vi "AUTO_HOME.vi"(8 "error in (no error)":errorcluster) -> (0 "error out":errorcluster)   [LabVIEW 2017]
doc: "This vi is for manually turn ON and OFF also monitor Output of PLCS. So this is manual screen."
uses:
  <vilib>/Utility/miscctls.llb/LVRowAndColumnUnsignedTypeDef.ctl
  8ff177a1-7a64-42a7-ac4f-5dbd57cfe52d.vi
  b56ad881-f772-481a-9ad8-33fdffb2c092.vi
  Global/PLC_to_Auto.vi
  <vilib>/Utility/file.llb/Read Delimited Spreadsheet (string).vi
  <vilib>/Utility/file.llb/Write Delimited Spreadsheet (string).vi
panel:
  out "Table":string[][](table)
  out "CYCLE STATUS 9":bool
  out "AUTO\nHOME STOP":bool
  in  "SPRING ABORT":bool
  in  "SPRING ACK":bool
  out "PART OK":bool
  out "SYSTEM READY":bool
  out "HAUSING STATUS":bool
  out "MAGNETIC STATUS":bool
  out "CBCT STATUS":bool
  out "PMR STATUS":bool
  out "KINEMATIC STATUS":bool
  out "KITTING ST NG COUNTER":u16 format="NG COUNTER: %.0f"
  out "KITTING ST OK COUNTER":u16 format="OK COUNTER: %.0f"
  out "KITTING ST CYCLE TIME":dbl format="CYCLE TIME : %.1f SEC"
  out "CYCLE STATUS 10":bool
  out "CYCLE STATUS 8":bool
  out "CYCLE STATUS 4":bool
  out "CYCLE STATUS 7":bool
  out "CYCLE STATUS 3":bool
  out "CYCLE STATUS 6":bool
  out "CYCLE STATUS 2":bool
  out "CYCLE STATUS 5":bool
  out "CYCLE STATUS 1":bool
  out "CYCLE TIME IN SEC":T1 {"CYCLE TIME 28" format="%.2f"; "CYCLE TIME 10" format="%.2f"; "CYCLE TIME 8" format="%.2f"; "CYCLE TIME 4" format="%.2f"; "CYCLE TIME 7" format="%.2f"; "CYCLE TIME 3" format="%.2f"; "CYCLE TIME 6" format="%.2f"; "CYCLE TIME 2" format="%.2f"; "CYCLE TIME 5" format="%.2f"; "CYCLE TIME 1" format="%.2f"}
  out "Plan Selected:":string
  out "USER:-":string
  out "ALARM Indicator":string
  out "DATE/TIME":string
  in  "Back":bool
  # "KITTING STATION - RCBO 2P2M"
  # "4.NEUTRAL\nIA ASSEMBLY"
  # "9.RIVITING\nSTATION"
  # "8.NEUTRAL\n2C ASSEMBLY"
  # "7.NEUTRAL\n2B ASSEMBLY"
  # "6.NEUTRAL\n2A ASSEMBLY"
  # "5.NEUTRAL\nIB ASSEMBLY"
  # "3.PHASE SIDE\nII ASSEMBLY"
  # "10.FINAL\nVISION SYSTEM"
  # "2.PHASE SIDE\nI ASSEMBLY"
  # "1.KITTING \nSTATION"
  # "CYCLE TIME IN SEC"
  # "OK COUNTER"
  # "NG COUNTER"
  # "CYCLE STATUS"
  # "ALARM:-"
  # "STATUS OF\n KITTING STATION"
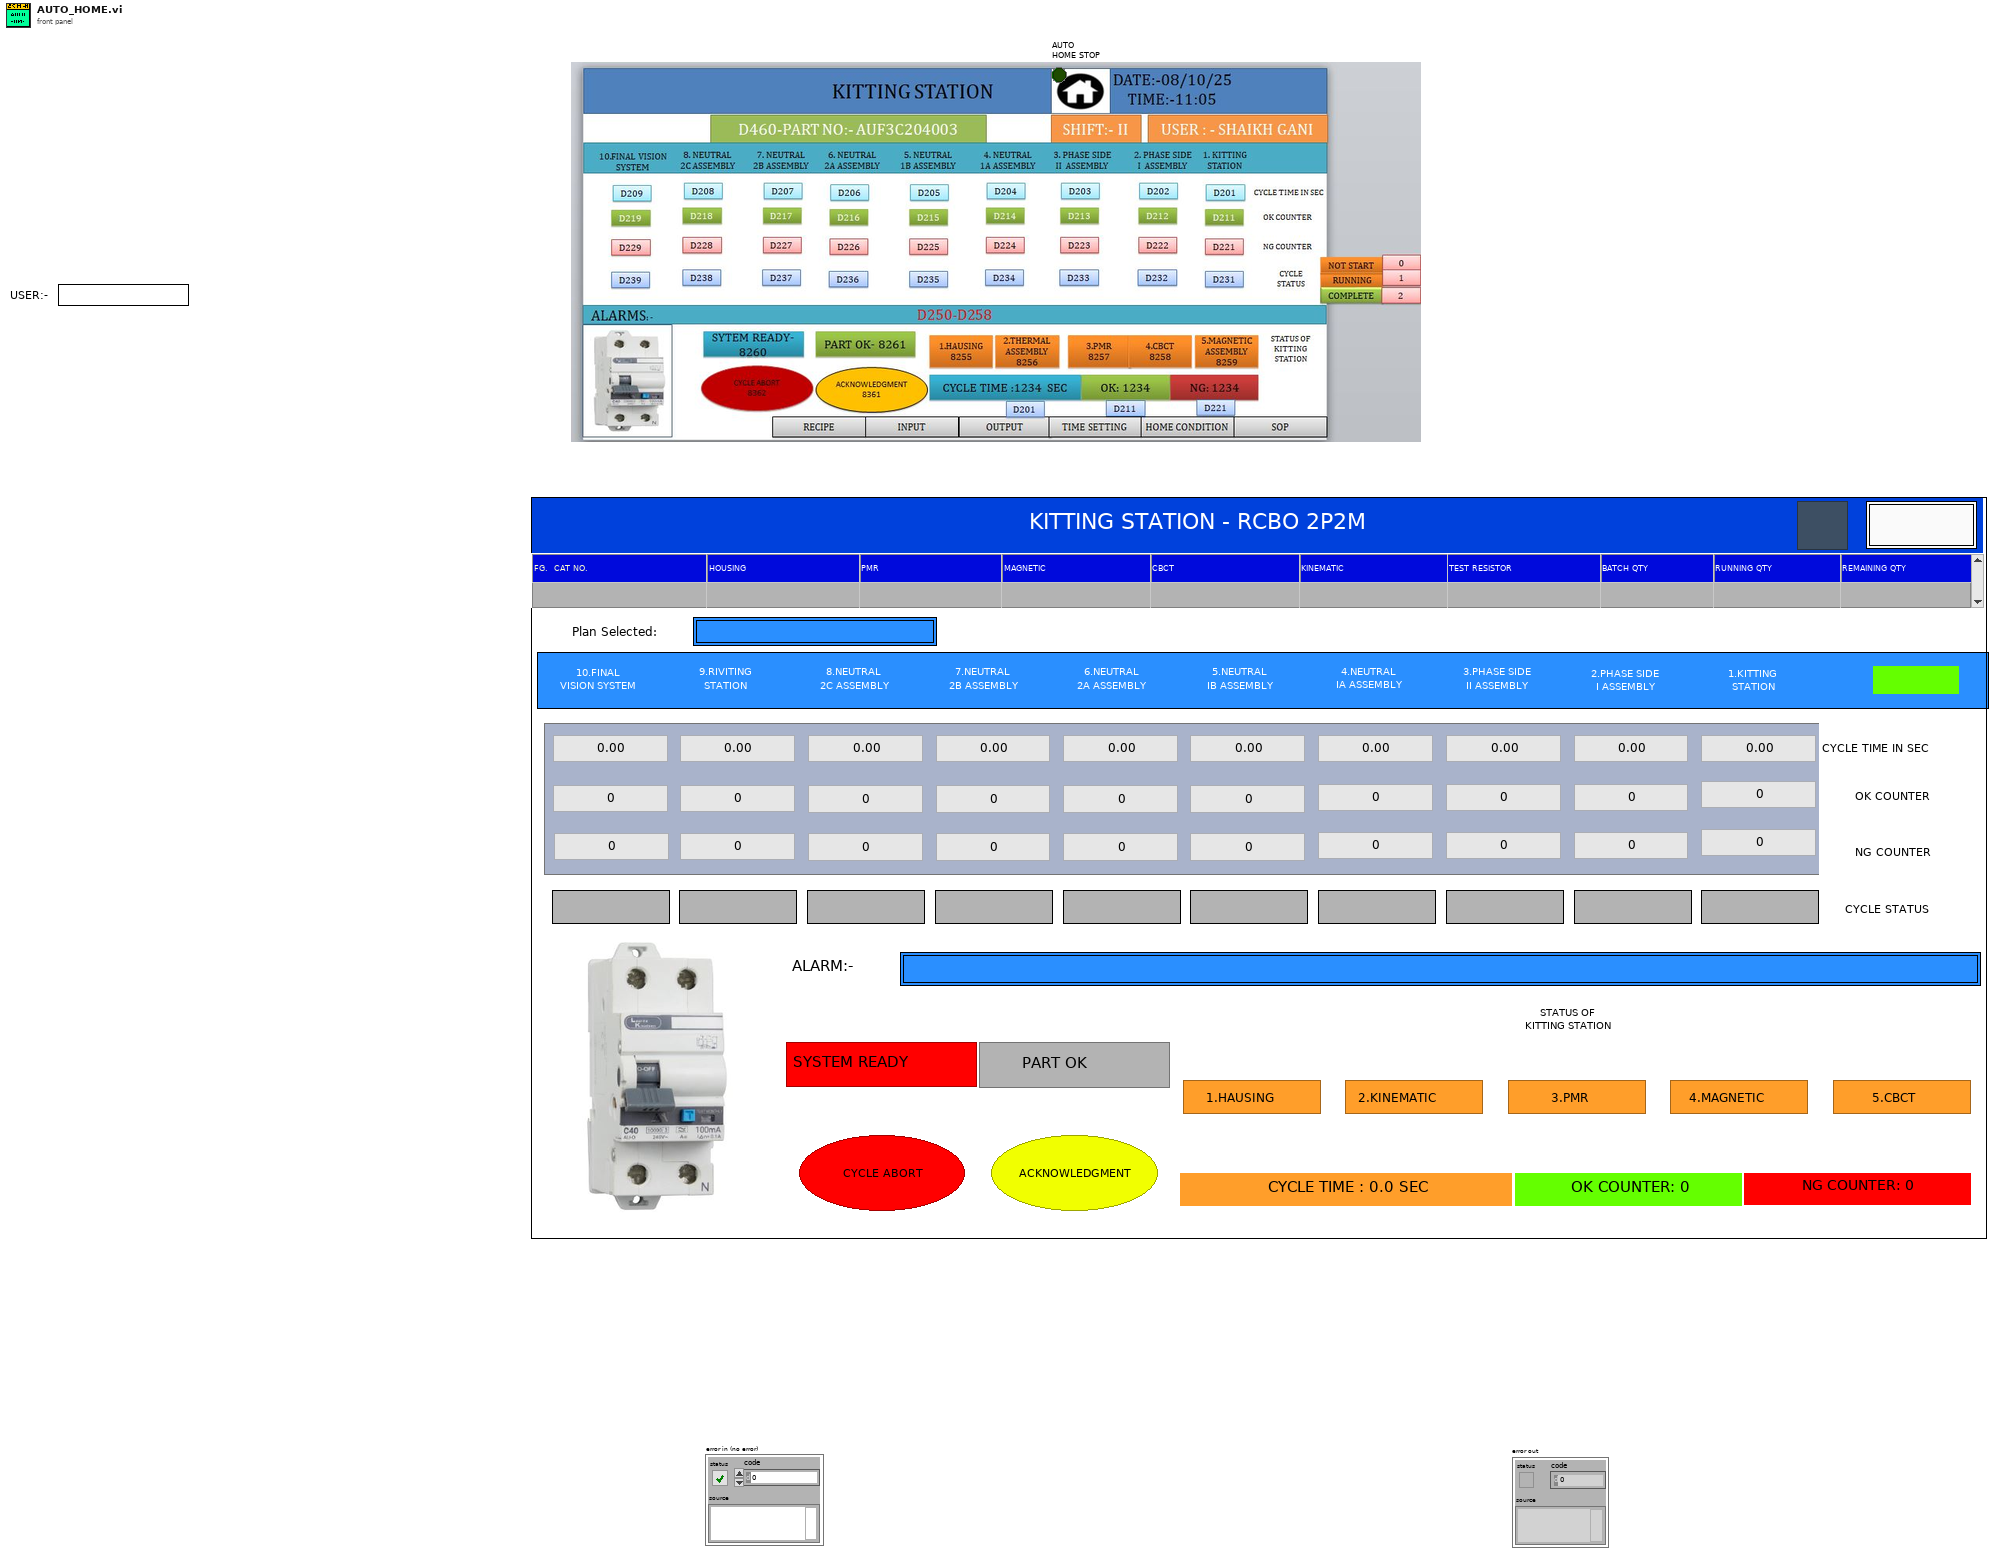
[diagram p1: front panel]
types:
  T1 = cluster{"[0]":dbl, "[1]":dbl, "[2]":dbl, "[3]":dbl, "[4]":dbl, "[5]":dbl, "[6]":dbl, "[7]":dbl, "[8]":dbl, "[9]":dbl, "CYCLE TIME 9":u16, "CYCLE TIME 12":u16, "CYCLE TIME 14":u16, "CYCLE TIME 16":u16, "CYCLE TIME 11":u16, "CYCLE TIME 13":u16, "CYCLE TIME 15":u16, "CYCLE TIME 17":u16, "CYCLE TIME 29":u16, "CYCLE TIME 18":u16, "CYCLE TIME 19":u16, "CYCLE TIME 21":u16, "CYCLE TIME 23":u16, "CYCLE TIME 25":u16, "CYCLE TIME 20":u16, "CYCLE TIME 22":u16, "CYCLE TIME 24":u16, "CYCLE TIME 26":u16, "CYCLE TIME 30":u16, "CYCLE TIME 27":u16}
  T2 = cluster{"SELECTED RECIPE":cluster{"TABLE":string[]}}
  T3 = typedef "LVRowAndColumnUnsignedTypeDef.ctl" = cluster{"Row":u32, "Column":u32}
  T4 = enum32{"invalid app kind", "Development System", "Run Time System", "Student Edition", "Embedded LabVIEW", "Evaluation", "Custom"}
  T5 = cluster{"[0]":dbl, "[1]":dbl, "[2]":dbl, "[3]":dbl, "[4]":dbl, "[5]":dbl, "[6]":dbl, "[7]":dbl, "[8]":dbl, "[9]":dbl, "[10]":dbl, "[11]":dbl, "[12]":dbl, "[13]":dbl, "[14]":dbl, "[15]":dbl, "[16]":dbl, "[17]":dbl, "[18]":dbl, "[19]":dbl, "[20]":dbl, "[21]":dbl, "[22]":dbl, "[23]":dbl, "[24]":dbl, "[25]":dbl, "[26]":dbl, "[27]":dbl, "[28]":dbl, "[29]":dbl}
  T6 = enum32{"Invalid", "Standard", "Closed", "Hidden", "Minimized", "Maximized"}
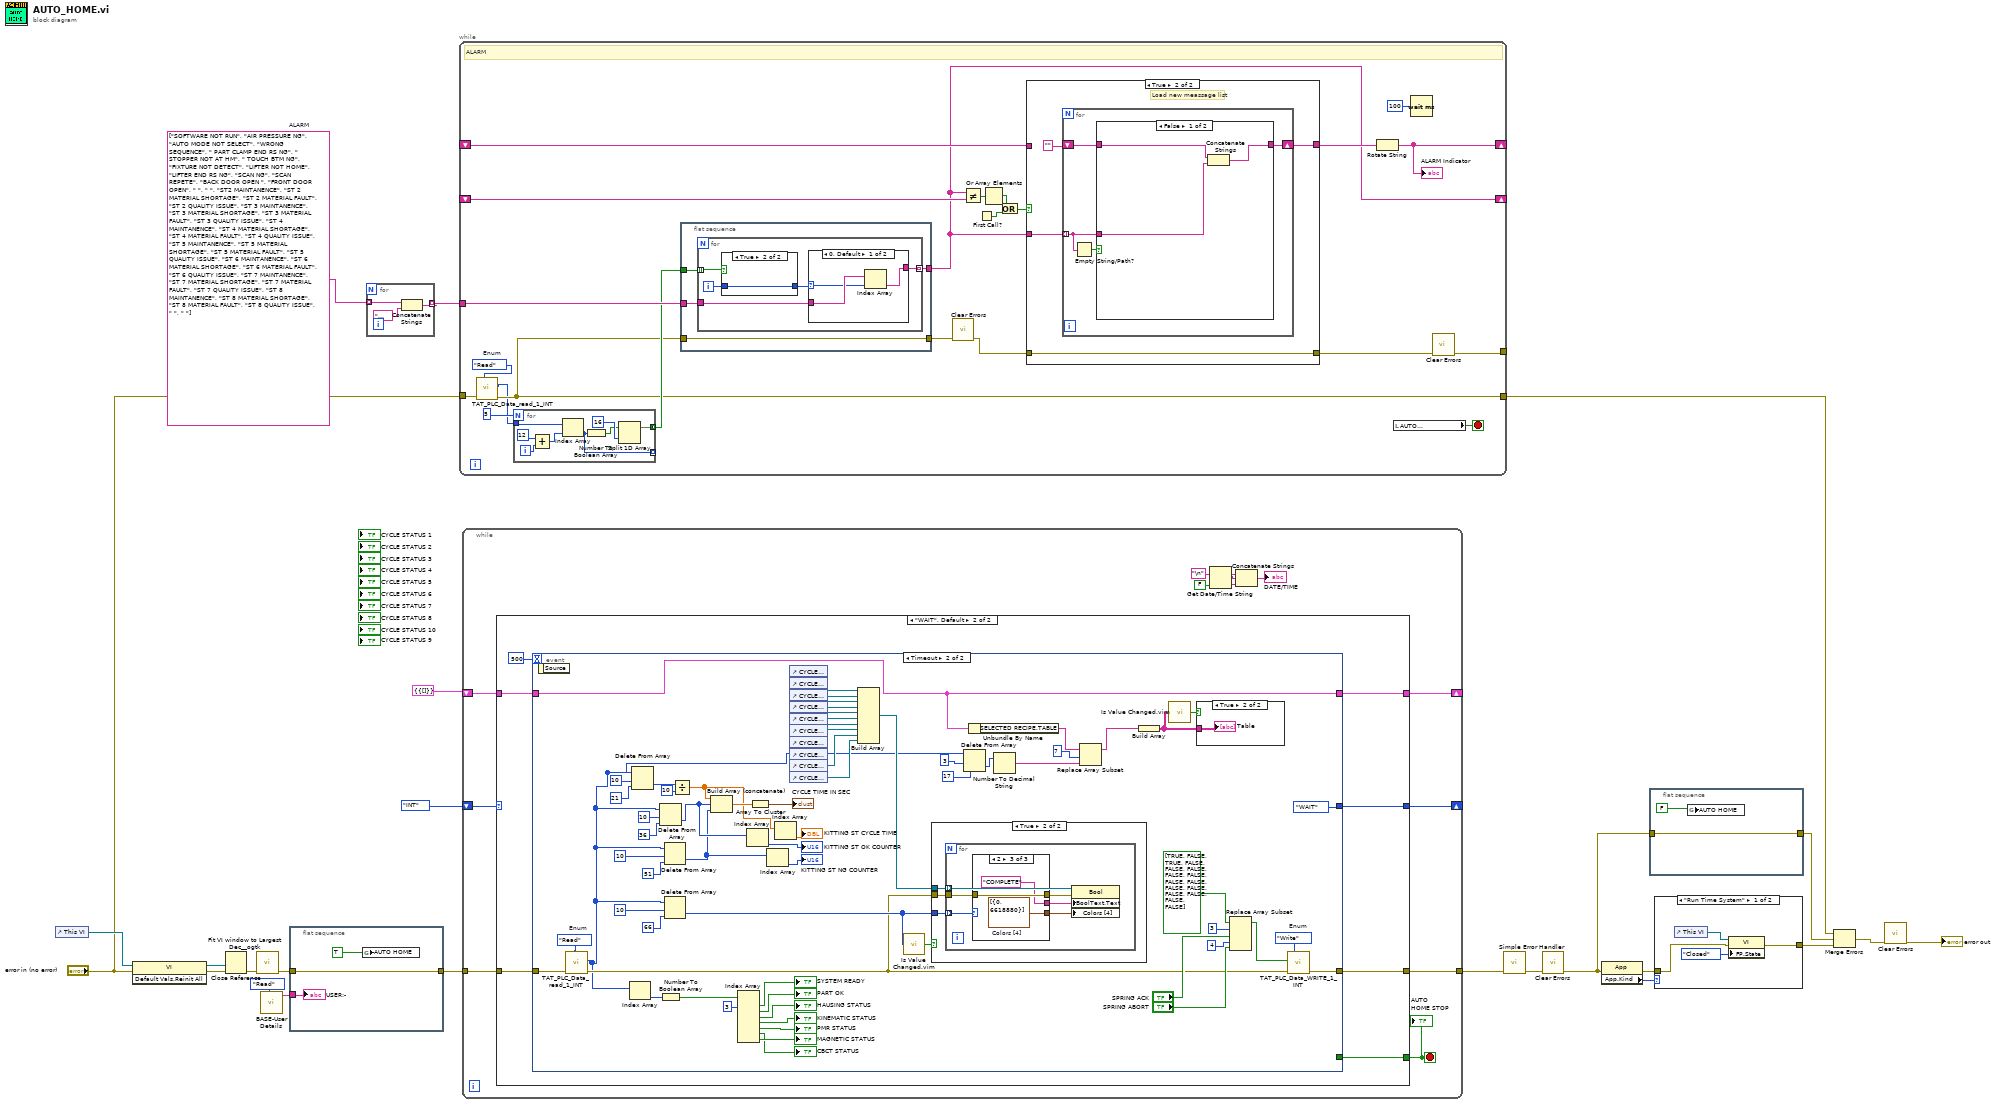
[diagram p0: block diagram]
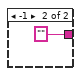
[diagram p2: hidden frame]
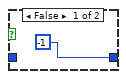
[diagram p3: hidden frame]
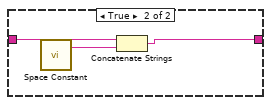
[diagram p5: hidden frame]
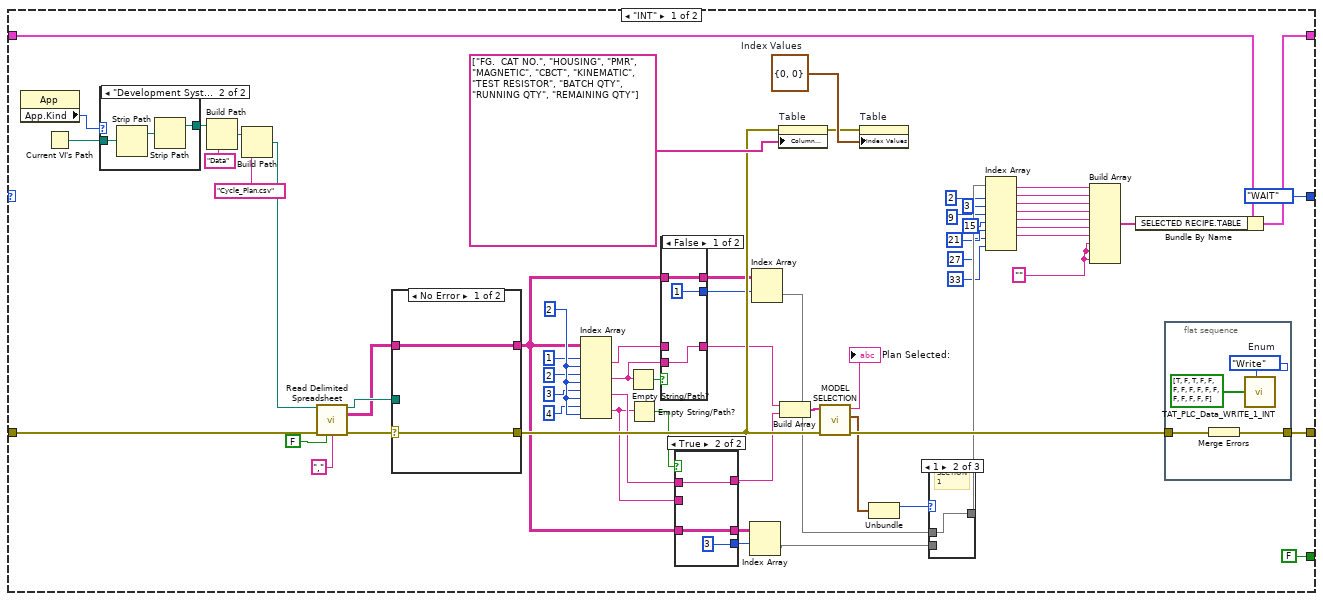
[diagram p7: hidden frame]
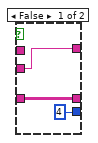
[diagram p10: hidden frame]
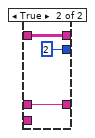
[diagram p11: hidden frame]
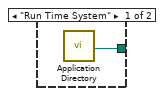
[diagram p12: hidden frame]
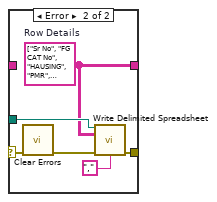
[diagram p13: hidden frame]
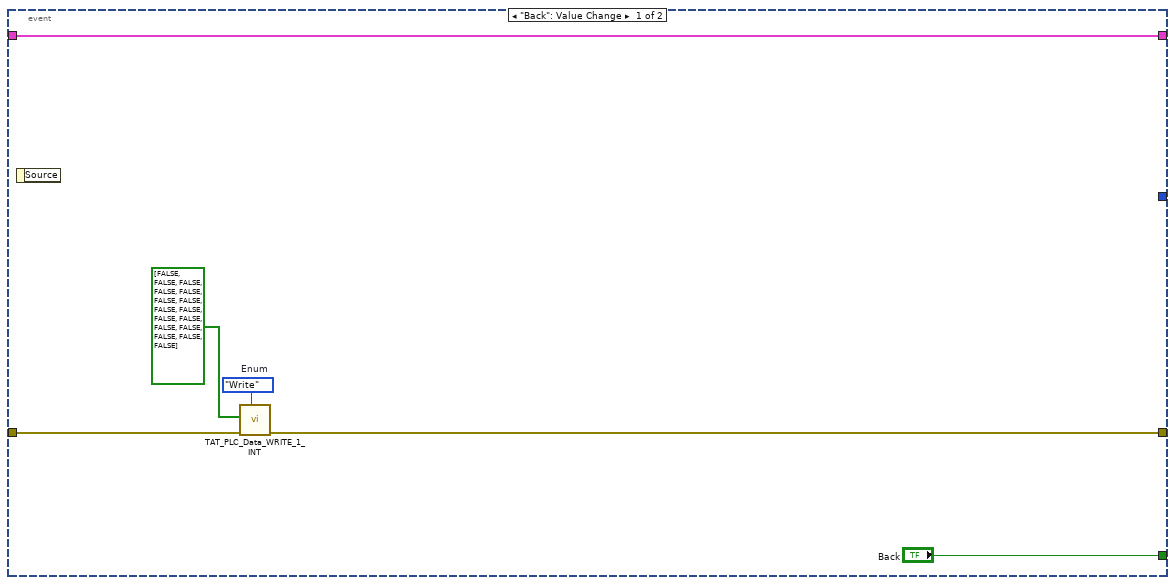
[diagram p14: hidden frame]
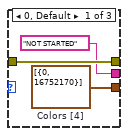
[diagram p17: hidden frame]
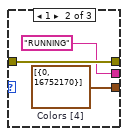
[diagram p18: hidden frame]
diagram:
  w2 = string[] ["SOFTWARE NOT RUN", "AIR PRESSURE NG", "AUTO MODE NOT SELECT", "WRONG SEQUENCE", " PART CLAMP END RS NG", " STOPPER NOT AT HM", " TOUCH BTM NG", "FIXTURE NOT DETECT", "LIFTER NOT HOME", "LIFTER END RS NG", "SCAN NG", "SCAN  REPETE", "BACK DOOR OPEN ", "FRONT DOOR OPEN", " ", " ", "ST2 MAINTANENCE", "ST 2 MATERIAL SHORTAGE", "ST 2 MATERIAL FAULT", "ST 2 QUALITY ISSUE", "ST 3 MAINTANENCE", "ST 3 MATERIAL SHORTAGE", "ST 3 MATERIAL FAULT", "ST 3 QUALITY ISSUE", "ST 4 MAINTANENCE", "ST 4 MATERIAL SHORTAGE", "ST 4 MATERIAL FAULT", "ST 4 QUALITY ISSUE", "ST 5 MAINTANENCE", "ST 5 MATERIAL SHORTAGE", "ST 5 MATERIAL FAULT", "ST 5 QUALITY ISSUE", "ST 6 MAINTANENCE", "ST 6 MATERIAL SHORTAGE", "ST 6 MATERIAL FAULT", "ST 6 QUALITY ISSUE", "ST 7 MAINTANENCE", "ST 7 MATERIAL SHORTAGE", "ST 7 MATERIAL FAULT", "ST 7 QUALITY ISSUE", "ST 8 MAINTANENCE", "ST 8 MATERIAL SHORTAGE", "ST 8 MATERIAL FAULT", "ST 8 QUALITY ISSUE", " ", " "]  # ALARM
  n1 = control-ref of="This VI"() -> (w19:refnum<vi>)
  n2 = invoke class="VI" method="Default Vals.Reinit All"(reference=w19, error in="error in (no error)") -> (reference out=w18:refnum<vi>, error out=w17:errorcluster)  [unwired: 1 in, 1 out]
  n3 = Close Reference(reference=w18, error in (no error)=w17) -> (error out=w16:errorcluster)
  n4 = call <userlib>:"Fit VI window to Largest Dec__ogtk.vi"("error in (no error)"=w16) -> ("error out"=w15:errorcluster)  [unwired: 5 in, 1 out]
  n5 = call "BASE-User Details.vi"("Enum"=enum16{"Read", "Write"}."Read") -> ("User Name Out"=w7:string)  [unwired: 9 in, 1 out]
  n6 = flat-sequence {
    tunnel: w15 -> [w26]
    tunnel: [w26] -> w11
    tunnel: w7 -> [w24]
    frame #0 {
      n7 = global write "PLC_to_Auto.vi" "AUTO HOME"(TRUE) -> ()
      "USER:-" <- w24
    }
  }
  n8 = for {
    tunnel: w2 -> [w29] mode=indexing
    tunnel: [w27] -> w5 mode=indexing
    n9 = Concatenate Strings(w29, "          ") -> (w27:string)
  }
  n10 = while {
    tunnel: "error in (no error)" -> [w33]
    tunnel: [w40] -> _
    tunnel: w5 -> [w38]
    shift-right: [w36] -> _
    shift-left: _ -> [w47]
    shift-right: [w46] -> _
    shift-left: _ -> [w48]
    tunnel: [w32] -> w3
    stop <- w37 stop-if-true
    w30 = enum16{"Read", "Write"}."Read"  # Enum
    # "ALARM"
    n11 = call "TAT_PLC_Data_read_1_INT.vi"("Enum"=w30, "error in (no error)"=w33) -> ("error out"=w32:errorcluster, "Array 2"=w31:u16[])  [unwired: 8 in]
    n12 = for {
      N: 5 -> [_]
      tunnel: w31 -> [w59]
      tunnel: [w53] -> w34 mode=concatenating
      tunnel: [w52] -> _ mode=indexing
      i -> [w57]
      n13 = Add(x=12, y=w57) -> (x+y=w56:i32)
      n14 = Index Array(array=w59, index=w56) -> (element=w52:u16)
      n15 = Number To Boolean Array(number=w52) -> (Boolean array=w54:bool[])
      n16 = Split 1D Array(array=w54, index=16) -> (first subarray=w53:bool[])  [unwired: 1 out]
    }
    n17 = flat-sequence {
      tunnel: [w61] -> w42
      tunnel: [w63] -> w46
      tunnel: w38 -> [w62]
      tunnel: w32 -> [w61]
      tunnel: w34 -> [w60]
      frame #0 {
        n18 = for {
          tunnel: w60 -> [w68] mode=indexing
          tunnel: [w64] -> w63 mode=indexing
          tunnel: w62 -> [w66]
          i -> [w67]
          n19 = case shown="True" w68 {
            tunnel: w67 -> [_ w74]
            tunnel: [-1 w74] -> w65
            frame False {
            }
            frame True {
            }
          }
          n20 = case shown="0, Default" w65 {
            selector: w65 -> [w70 _]
            tunnel: w66 -> [w71 _]
            tunnel: [w69 ""] -> w64
            frame 0, Default {
              n21 = Index Array(array=w71, index=w70) -> (element=w69:string)
            }
            frame -1 {
            }
          }
        }
      }
    }
    n22 = call <vilib>:"Clear Errors.vi"("error in (no error)"=w42) -> ("error out"=w41:errorcluster)  [unwired: 5 in, 1 out]
    n23 = Not Equal?(x=w46, y=w48) -> (x != y?=w50:bool[])
    n24 = First Call?() -> (First Call?: T/F=w45:bool)
    n25 = Or Array Elements(Boolean array=w50) -> (logical OR=w44:bool)
    n26 = Or(x=w44, y=w45) -> (x .or. y?=w43:bool)
    n27 = case shown="True" w43 {
      tunnel: [w76 w78] -> w49
      tunnel: w47 -> [w76 _]
      tunnel: w46 -> [_ w79]
      tunnel: w41 -> [w75 w77]
      tunnel: [w75 w77] -> w39
      frame False {
      }
      frame True {
        # "Load new meassage list"
        n28 = for {
          tunnel: w79 -> [w82] mode=indexing
          shift-right: [w84] -> w78
          shift-left: "" -> [w83]
          n29 = Empty String/Path?(string/path=w82) -> (empty?=w81:bool)
          n30 = case shown="False" w81 {
            tunnel: [w87 w90] -> w84
            tunnel: w83 -> [w86 w89]
            tunnel: w82 -> [w85 _]
            frame False {
              n31 = Concatenate Strings(w86, w85) -> (w87:string)
            }
            frame True {
              n32 = call <vilib>:"Space Constant.vi"() -> ("String"=w88:string)
              n33 = Concatenate Strings(w89, w88) -> (w90:string)
            }
          }
        }
      }
    }
    n34 = Rotate String(1:w49) -> (0:w36:string)
    "ALARM Indicator" <- w36
    n35 = local read "AUTO\nHOME STOP"() -> (w37:bool)
    n36 = Wait (ms)(milliseconds to wait=u32 100) -> ()  [unwired: 1 out]
    n37 = call <vilib>:"Clear Errors.vi"("error in (no error)"=w39) -> ("error out"=w40:errorcluster)  [unwired: 5 in, 1 out]
  }
  n38 = while {
    tunnel: w11 -> [w102]
    tunnel: [w101] -> w22
    shift-right: [w98] -> _
    shift-left: enum16{"INT", "WAIT"}."INT" -> [w99]
    shift-right: [w92] -> _
    shift-left: T2 {"SELECTED RECIPE"={"TABLE"=[]}} -> [w91]
    stop <- w100 stop-if-true
    n39 = case shown="\"WAIT\", Default" w99 {
      tunnel: w102 -> [w161 w203]
      tunnel: [w122 w202] -> w101
      tunnel: [FALSE w201] -> w100
      tunnel: [enum16{"INT", "WAIT"}."WAIT" w199] -> w98
      tunnel: [w104 w198] -> w92
      tunnel: w91 -> [w105 w197]
      frame "INT" {
        w113 = ""
        w146 = 2
        w148 = T3 {"Row"=0, "Column"=0}  # Index Values
        n40 = property class="App"() -> ("App.Kind"=w159:T4)  [unwired: 2 in, 2 out]
        n41 = Current VI's Path() -> (path=w160:path)
        n42 = case shown="\"Development System\", Default" w159 {
          tunnel: w160 -> [_ w187]
          tunnel: [w185 w186] -> w157
          frame "Run Time System" {
            n43 = call <vilib>:"Application Directory.vi"() -> ("Application Directory"=w185:path)
          }
          frame "Development System", Default {
            n44 = Strip Path(path=w187) -> (stripped path=w188:path)  [unwired: 1 out]
            n45 = Strip Path(path=w188) -> (stripped path=w186:path)  [unwired: 1 out]
          }
        }
        n46 = Build Path(base path=w157, name or relative path="Data") -> (appended path=w155:path)
        n47 = Build Path(base path=w155, name or relative path="Cycle_Plan.csv") -> (appended path=w154:path)
        n48 = call-poly <vilib>:"Read Delimited Spreadsheet.vi"("file path (dialog if empty)"=w154, "error in (no error)"=w161, "transpose? (F)"=FALSE, "delimiter (\\t)"=",") -> ("new file path (Not A Path if cancelled)"=w165:path, "all rows"=w164:string[][], "error out"=w166:errorcluster)  [unwired: 6 in, 3 out]
        n49 = case shown="No Error" w166 {
          selector: w166 -> [w190 w196]
          tunnel: [w190 w194] -> w149
          tunnel: w165 -> [_ w193]
          tunnel: [w189 w191] -> w126
          tunnel: w164 -> [w189 _]
          frame No Error {
          }
          frame Error {
            w191 = string[][] [["Sr No", "FG CAT No", "HAUSING", "PMR", "MAGNETIC ASLY", "CBCT GROUP", "KINEMATIC ASLY", "TEST RESISTOR"]]  # Row Details
            n50 = call <vilib>:"Clear Errors.vi"("error in (no error)"=w196) -> ("error out"=w195:errorcluster)  [unwired: 5 in, 1 out]
            n51 = call-poly <vilib>:"Write Delimited Spreadsheet.vi"("file path (dialog if empty)"=w193, "2D data"=w191, "error in (no error)"=w195, "delimiter (\\t)"=",") -> ("error out"=w194:errorcluster)  [unwired: 10 in, 1 out]
          }
        }
        n52 = Index Array(array=w126, index (row) #1=1, index (col) #1=w146, index (row) #2=2, index (col) #2=w146, index (row) #3=3, index (col) #3=w146, index (row) #4=4, index (col) #4=w146) -> (element #1=w140:string, element #2=w139:string, element #3=w137:string, element #4=w136:string)
        n53 = Empty String/Path?(string/path=w139) -> (empty?=w141:bool)
        n54 = Empty String/Path?(string/path=w136) -> (empty?=w138:bool)
        n55 = case shown="False" w141 {
          tunnel: w140 -> [_ w184]
          tunnel: w139 -> [w181 _]
          tunnel: [w181 w184] -> w135
          tunnel: w126 -> [w179 w183]
          tunnel: [1 2] -> w129
          tunnel: [w179 w183] -> w128
          frame False {
          }
          frame True {
          }
        }
        n56 = case shown="True" w138 {
          tunnel: w137 -> [_ w178]
          tunnel: w136 -> [w175 _]
          tunnel: [w175 w178] -> w130
          tunnel: w126 -> [w174 w176]
          tunnel: [w174 w176] -> w125
          tunnel: [4 3] -> w124
          frame False {
          }
          frame True {
          }
        }
        n57 = Index Array(array=w125, index (row)=w124) -> (element=w123:string[])  [unwired: 1 in]
        n58 = Index Array(array=w128, index (row)=w129) -> (element=w127:string[])  [unwired: 1 in]
        n59 = property on="Table" class="Tbl (strict)"(error in=w149, "Column Headers[]"=string[] ["FG.  CAT NO.", "HOUSING", "PMR", "MAGNETIC", "CBCT", "KINEMATIC", "TEST RESISTOR", "BATCH QTY", "RUNNING QTY", "REMAINING QTY"]) -> (error out=w147:errorcluster)  [unwired: 1 in, 1 out]
        n60 = Build Array(w135, w130) -> (w134:string[])
        n61 = call "MODEL SELECTION.vi"("error in (no error)"=w149, "Plan List"=w134) -> ("error out 2"=w152:errorcluster, "SELECTED RECIPE\nand COMBI OF BIN- INDEX"=w132:cluster{"RECIPE INDEX":i32, "COMBI BIN":i32}, "Plan Selected"=→"Plan Selected:":string)  [unwired: 7 in]
        n62 = property on="Table" class="Tbl (strict)"(error in=w147, "Index Values"=w148) -> ()  [unwired: 1 in, 2 out]
        n63 = Unbundle(w132) -> ("RECIPE INDEX"=w131:i32)  [unwired: 1 out]
        n64 = case shown="1" w131 {
          tunnel: w127 -> [_ w171 _]
          tunnel: w123 -> [_ _ w172]
          tunnel: [_ w171 w172] -> w121
          frame 0, Default {
          }
          frame 1 {
            # "SECTION 1"
          }
          frame 2 {
            # "SECTION 2"
          }
        }
        n65 = Index Array(array=w121, index #1=2, index #2=3, index #3=9, index #4=15, index #5=21, index #6=27, index #7=33) -> (element #1=w112:string, element #2=w111:string, element #3=w110:string, element #4=w109:string, element #5=w108:string, element #6=w107:string, element #7=w106:string)
        n66 = Build Array(w112, w111, w110, w109, w108, w107, w106, w113, w113, w113) -> (w103:string[])
        n67 = Bundle By Name(cluster=w105, "SELECTED RECIPE.TABLE"=w103) -> (w104:T2)
        n68 = flat-sequence {
          tunnel: w152 -> [w170]
          tunnel: [w169] -> w122
          frame #0 {
            w168 = enum16{"Read", "Write"}."Write"  # Enum
            n69 = Merge Errors(w170) -> (w169:errorcluster)
            n70 = call "TAT_PLC_Data_WRITE_1_INT.vi"("Enum"=w168, "Array"=bool[] [TRUE, FALSE, TRUE, FALSE, FALSE, FALSE, FALSE, FALSE, FALSE, FALSE, FALSE, FALSE, FALSE, FALSE, FALSE, FALSE]) -> ()  [unwired: 8 in, 2 out]
          }
        }
      }
      frame "WAIT", Default {
        n71 = event shown="[1] Timeout" {
          selector: _ -> [_ _]
          dyn-events: _ -> [_ _]
          timeout: 500 -> [_ _]
          tunnel: w203 -> [w206 w230]
          tunnel: [w205 w245] -> w202
          tunnel: ["Back" _] -> w201
          tunnel: [_ enum16{"INT", "WAIT"}."WAIT"] -> w199
          tunnel: [w204 w228] -> w198
          tunnel: w197 -> [w204 w228]
          event "Back": Value Change {
            w208 = enum16{"Read", "Write"}."Write"  # Enum
            n72 = event-data() -> ()  [unwired: 1 in, 1 out]
            n73 = call "TAT_PLC_Data_WRITE_1_INT.vi"("Enum"=w208, "error in (no error)"=w206, "Array"=bool[] [FALSE, FALSE, FALSE, FALSE, FALSE, FALSE, FALSE, FALSE, FALSE, FALSE, FALSE, FALSE, FALSE, FALSE, FALSE, FALSE]) -> ("error out"=w205:errorcluster)  [unwired: 7 in, 1 out]
          }
          event Timeout {
            w244 = enum16{"Read", "Write"}."Write"  # Enum
            w231 = enum16{"Read", "Write"}."Read"  # Enum
            n74 = event-data() -> ()  [unwired: 1 in, 1 out]
            n75 = call "TAT_PLC_Data_read_1_INT.vi"("Enum"=w231, "error in (no error)"=w230) -> ("error out"=w229:errorcluster, "Array 2"=w217:u16[])  [unwired: 8 in]
            n76 = Index Array(array=w217) -> (element=w232:u16)  [unwired: 1 in]
            n77 = Delete From Array(array=w217, length=10 ("index"), index=21) -> (deleted portion=w235:u16[])  [unwired: 1 out]
            n78 = Delete From Array(array=w217, length=10 ("index"), index=36) -> (deleted portion=w249:u16[])  [unwired: 1 out]
            n79 = Number To Boolean Array(number=w232) -> (Boolean array=w233:bool[])
            n80 = Delete From Array(array=w217, length=10 ("index"), index=51) -> (deleted portion=w248:u16[])  [unwired: 1 out]
            n81 = Delete From Array(array=w217, length=10 ("index"), index=66) -> (deleted portion=w253:u16[])  [unwired: 1 out]
            n82 = Divide(x=w235, y=10 ("index")) -> (x/y=w234:dbl[])
            n83 = Build Array (concatenate)(w234, w249, w248) -> (w269:dbl[])
            n84 = Index Array(array=w233, index #1=3) -> (element #1=→"SYSTEM READY":bool, element #2=→"PART OK":bool, element #3=→"HAUSING STATUS":bool, element #4=→"KINEMATIC STATUS":bool, element #5=→"PMR STATUS":bool, element #6=→"MAGNETIC STATUS":bool, element #7=→"CBCT STATUS":bool)  [unwired: 6 in]
            n85 = Index Array(array=w249) -> (element=→"KITTING ST OK COUNTER":u16)  [unwired: 1 in]
            n86 = Array To Cluster(array=w269) -> (cluster=→"CYCLE TIME IN SEC":T5)
            n87 = Index Array(array=w248) -> (element=→"KITTING ST NG COUNTER":u16)  [unwired: 1 in]
            n88 = Index Array(array=w234) -> (element=→"KITTING ST CYCLE TIME":dbl)  [unwired: 1 in]
            n89 = control-ref of="CYCLE STATUS 1"() -> (w263:refnum<vi>)
            n90 = control-ref of="CYCLE STATUS 2"() -> (w262:refnum<vi>)
            n91 = control-ref of="CYCLE STATUS 3"() -> (w261:refnum<vi>)
            n92 = control-ref of="CYCLE STATUS 4"() -> (w260:refnum<vi>)
            n93 = control-ref of="CYCLE STATUS 5"() -> (w259:refnum<vi>)
            n94 = control-ref of="CYCLE STATUS 6"() -> (w258:refnum<vi>)
            n95 = control-ref of="CYCLE STATUS 7"() -> (w257:refnum<vi>)
            n96 = control-ref of="CYCLE STATUS 8"() -> (w256:refnum<vi>)
            n97 = control-ref of="CYCLE STATUS 9"() -> (w246:refnum<vi>)
            n98 = control-ref of="CYCLE STATUS 10"() -> (w247:refnum<vi>)
            n99 = Build Array(w263, w262, w261, w260, w259, w258, w257, w256, w246, w247) -> (w255:refnum<vi>[])
            n100 = call "Is Value Changed.vim"("value"=w253) -> ("changed or first call?"=w254:bool)
            n101 = case shown="True" w254 {
              tunnel: w255 -> [_ w277]
              tunnel: w253 -> [_ w276]
              tunnel: w229 -> [_ w275]
              frame False {
              }
              frame True {
                n102 = for {
                  tunnel: w277 -> [w283] mode=indexing
                  tunnel: w276 -> [w280] mode=indexing
                  tunnel: w275 -> [w282]
                  n103 = case shown="2" w280 {
                    tunnel: w282 -> [w286 w289 w292]
                    tunnel: [w286 w289 w292] -> w281
                    tunnel: [w285 w288 w291] -> w279
                    tunnel: ["NOT STARTED" "RUNNING" "COMPLETE"] -> w278
                    frame 0, Default {
                      w285 = cluster{u32, u32}[] [{0, 16752170}]  # Colors [4]
                    }
                    frame 1 {
                      w288 = cluster{u32, u32}[] [{0, 16752170}]  # Colors [4]
                    }
                    frame 2 {
                      w291 = cluster{u32, u32}[] [{0, 6618880}]  # Colors [4]
                    }
                  }
                  n104 = property class="Bool"(reference=w283, error in=w281, "BoolText.Text"=w278, "Colors [4]"=w279) -> ()  [unwired: 2 out]
                }
              }
            }
            n105 = Delete From Array(array=w217, length=3, index=17) -> (deleted portion=w214:u16[])  [unwired: 1 out]
            n106 = Unbundle By Name(w228) -> ("SELECTED RECIPE.TABLE"=w211:string[])
            n107 = Number To Decimal String(number=w214) -> (decimal integer string=w212:string[])  [unwired: 1 in]
            n108 = Replace Array Subset(array=w211, new element=w212, index=7) -> (w210:string[])
            n109 = Build Array(w210) -> (w219:string[][])
            n110 = call "Is Value Changed.vim"("value"=w219) -> ("changed or first call?"=w218:bool)
            n111 = case shown="True" w218 {
              tunnel: w219 -> [_ w274]
              frame False {
              }
              frame True {
                "Table" <- w274
              }
            }
            n112 = Replace Array Subset(array=bool[] [TRUE, FALSE, TRUE, FALSE, FALSE, FALSE, FALSE, FALSE, FALSE, FALSE, FALSE, FALSE, FALSE, FALSE, FALSE, FALSE], new element #1="SPRING ACK", index #1=3, new element #2="SPRING ABORT", index #2=4) -> (w238:bool[])
            n113 = call "TAT_PLC_Data_WRITE_1_INT.vi"("Enum"=w244, "error in (no error)"=w229, "Array"=w238) -> ("error out"=w245:errorcluster)  [unwired: 7 in, 1 out]
          }
        }
      }
    }
    "AUTO\nHOME STOP" <- w100
    n114 = Get Date/Time String(want seconds? (F)=FALSE) -> (date string=w97:string, time string=w96:string)  [unwired: 2 in]
    n115 = Concatenate Strings(w97, "\n", w96) -> (→"DATE/TIME":string)
  }
  n116 = call <vilib>:"Simple Error Handler.vi"("error in (no error)"=w22) -> ("error out"=w14:errorcluster)  [unwired: 4 in, 4 out]
  n117 = call <vilib>:"Clear Errors.vi"("error in (no error)"=w14) -> ("error out"=w10:errorcluster)  [unwired: 5 in, 1 out]
  n118 = property class="App"(error in=w10) -> (error out=w12:errorcluster, "App.Kind"=w13:T4)  [unwired: 1 in, 1 out]
  n119 = flat-sequence {
    tunnel: w10 -> [w294]
    tunnel: [w294] -> w9
    frame #0 {
      n120 = global write "PLC_to_Auto.vi" "AUTO HOME"(FALSE) -> ()
    }
  }
  n121 = case shown="\"Run Time System\"" w13 {
    tunnel: w12 -> [w296 w299]
    tunnel: [w295 w299] -> w20
    frame "Run Time System" {
      n122 = control-ref of="This VI"() -> (w298:refnum<vi>)
      n123 = property class="VI"(reference=w298, error in=w296, "FP.State"=T6."Closed" ("Front Panel Window:State")) -> (error out=w295:errorcluster)  [unwired: 1 out]
    }
    frame "Development System", Default {
    }
  }
  n124 = Merge Errors(w3, w9, w20) -> (w21:errorcluster)
  n125 = call <vilib>:"Clear Errors.vi"("error in (no error)"=w21) -> ("error out"=→"error out":errorcluster)  [unwired: 5 in, 1 out]
